vi "SLM_GenerateHologram.vi"(0 "x angle (mrad)":dbl, 1 "y angle (mrad)":dbl, 2 "LUT":dbl[](array[numeric]), 3 "beam parameters":T1={"amplitudeMatrix"=[], "SLM width (m)"=0.01498, "SLM height (m)"=0.01092, "wavelength (m)"=6.33e-07, "Resolution x"=1920, "Resolution y"=1080} {"Resolution x" format="%#.0f"; "SLM width (m)" format="%_6f"; "SLM height (m)" format="%#_6f"}, 4 "Masking":bool) -> (5 "Hologram":dbl[][](array[numeric]))   [LabVIEW 2024]
uses:
  typeDefs/BPandSLM.ctl
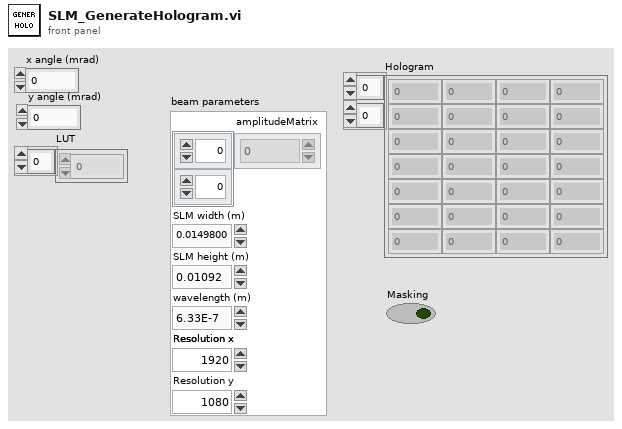
[diagram p1: front panel]
types:
  T1 = typedef "BPandSLM.ctl" = cluster{"amplitudeMatrix":csg[][], "SLM width (m)":dbl, "SLM height (m)":dbl, "wavelength (m)":dbl, "Resolution x":u32, "Resolution y":u32}
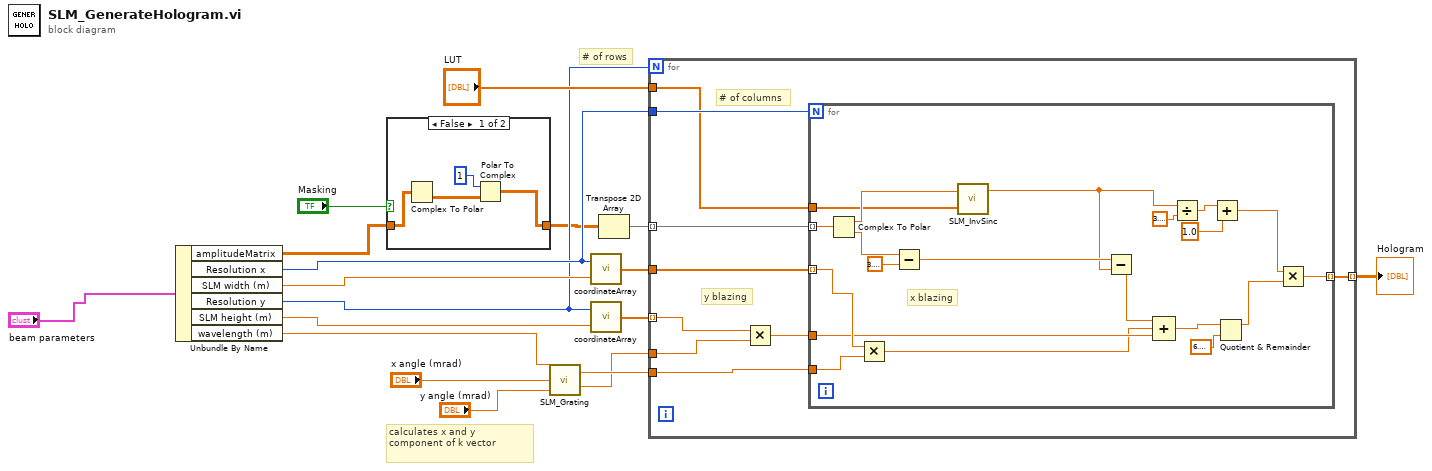
[diagram p0: block diagram]
diagram:
  # "calculates x and y \ncomponent of k vector"
  # "# of columns"
  # "# of rows"
  # "# of rows"
  n1 = Unbundle By Name("beam parameters") -> ("amplitudeMatrix"=w6:csg[][], "Resolution x"=w5:u32, "SLM width (m)"=w17:dbl, "Resolution y"=w4:u32, "SLM height (m)"=w16:dbl, "wavelength (m)"=w15:dbl)
  n2 = case shown="False" "Masking" {
    tunnel: w6 -> [w22 w23]
    tunnel: [w19 w23] -> w3
    frame False {
      n3 = Complex To Polar(r * e^(i*theta)=w22) -> (theta=w21:sgl[][])  [unwired: 1 out]
      n4 = Polar To Complex(1:w21, 2:1) -> (0:w19:csg[][])
    }
    frame True {
    }
  }
  n5 = call "SLM_Grating.vi"("y angle (mrad)"="y angle (mrad)", "x angle (mrad)"="x angle (mrad)", "wavelength"=w15) -> ("k y"=w8:dbl, "k x"=w11:dbl)
  n6 = call "coordinateArray.vi"("width of represented x (or y) range (in m; default 1E-3=1mm)"=w17, "array size (default 64)"=w5) -> ("x array"=w12:sgl[])
  n7 = call "coordinateArray.vi"("width of represented x (or y) range (in m; default 1E-3=1mm)"=w16, "array size (default 64)"=w4) -> ("x array"=w10:sgl[])
  n8 = Transpose 2D Array(2D array=w3) -> (transposed array=w2:csg[][])
  n9 = for {
    N: w4 -> [_]
    tunnel: w2 -> [w32] mode=indexing
    tunnel: w11 -> [w31]
    tunnel: [w30] -> w18 mode=indexing
    tunnel: w5 -> [w29]
    tunnel: w12 -> [w28]
    tunnel: w10 -> [w27] mode=indexing
    tunnel: w8 -> [w25]
    tunnel: "LUT" -> [w26]
    # "y blazing"
    n10 = Multiply(x=w27, y=w25) -> (x*y=w24:dbl)
    n11 = for {
      N: w29 -> [_]
      tunnel: w32 -> [w52] mode=indexing
      tunnel: w31 -> [w34]
      tunnel: [w39] -> w30 mode=indexing
      tunnel: w28 -> [w38] mode=indexing
      tunnel: w24 -> [w37]
      tunnel: w26 -> [w35]
      # "x blazing"
      n12 = Complex To Polar(r * e^(i*theta)=w52) -> (r=w45:sgl, theta=w48:sgl)
      n13 = Multiply(x=w38, y=w34) -> (x*y=w33:dbl)
      n14 = Subtract(x=w48, y=3.141592653589793) -> (x-y=w46:dbl)
      n15 = call "SLM_InvSinc.vi"("LUT"=w35, "Argument"=w45) -> ("InvSinc"=w36:dbl)
      n16 = Subtract(x=w46, y=w36) -> (x-y=w44:dbl)
      n17 = Compound Arithmetic op=ADD(w44, w33, w37) -> (w43:dbl)
      n18 = Divide(x=w36, y=3.141592653589793) -> (x/y=w50:dbl)
      n19 = Add(x=w50, y=1.0) -> (x+y=w41:dbl)
      n20 = Quotient & Remainder(x=w43, y=6.283185307179586) -> (x-y*floor(x/y)=w40:dbl)  [unwired: 1 out]
      n21 = Multiply(x=w41, y=w40) -> (x*y=w39:dbl)
    }
  }
  "Hologram" <- w18
